vi "PH_Powermeter_BaseClass.set State.vi"(0 "VI in":refnum<vi>, 2 "State":T1, 5 "error in (no error)":errorcluster) -> (14 "VI out":refnum<vi>, 19 "error out":errorcluster)   [LabVIEW 2014, in "PH_Powermeter_BaseClass.lvlib"]
uses:
  PH_Powermeter_BaseClass.lvlib
  PH_Powermeter_BaseClass.State.ctl
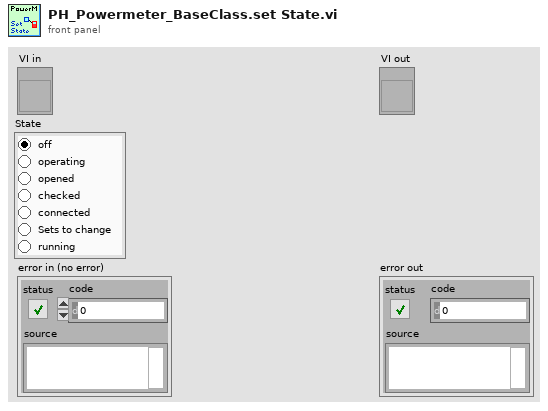
[diagram p1: front panel]
types:
  T1 = typedef "PH_Powermeter_BaseClass.lvlib/PH_Powermeter_BaseClass.State.ctl" = enum32{"off", "operating", "opened", "checked", "connected", "Sets to change", "running"}
  T2 = typedef "PH_Powermeter_BaseClass.lvlib/PH_Powermeter_BaseClass.i attribute.ctl" = cluster{"GUI References":T3, "Connection":T4, "Head Attributes":T5, "VISA resource":refnum<visa-resource-name>, "Energy":T6, "Service ID Energy":i32, "Wanted Settings":T7, "Current Settings":T7}
  T3 = typedef "PH_Powermeter_BaseClass.lvlib/PH_Powermeter_BaseClass.GUI Refs.ctl" = cluster{"Head Attributes":refnum<vi>, "Energy":refnum<vi>, "Connection":refnum<vi>, "VISA Resource":refnum<vi>, "Scaling Factor":refnum<vi>, "Range":refnum<vi>, "Wavelength":refnum<vi>, "Trigger Level":refnum<vi>, "Wanted Settings":refnum<vi>, "Current Settings":refnum<vi>}
  T4 = typedef "PH_Powermeter_BaseClass.lvlib/PH_Powermeter_BaseClass.Connection.ctl" = cluster{"failed checks":i8, "Timeout":bool, "Data read":string, "Failure":bool, "Error":bool, "State":T1}
  T5 = typedef "PH_Powermeter_BaseClass.lvlib/PH_Powermeter_BaseClass.Head Attributes.ctl" = cluster{"Instrument Type":string, "Head Version":string, "Head Name":string, "Serial Number":string, "Firmware":string, "Sensor Type":string, "MinimumRange":u32, "Maximum Range":u32, "Min Wavelength":i32, "Max Wavelength":i32}
  T6 = typedef "PH_Powermeter_BaseClass.lvlib/PH_Powermeter_BaseClass.Energy.ctl" = cluster{"current Value":dbl, "unscaled":dbl, "Scaling Factor":dbl}
  T7 = typedef "PH_Powermeter_BaseClass.lvlib/PH_gentec_BaseClass.Head Settings.ctl" = cluster{"Trigger Level":dbl, "Wavelength":u32, "Range":u32}
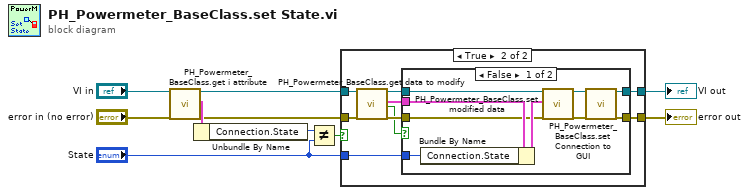
[diagram p0: block diagram]
diagram:
  n1 = call "PH_Powermeter_BaseClass.get i attribute.vi"("i ref in"="VI in", "error in (no error)"="error in (no error)") -> ("i ref out"=w1:refnum<vi>, "i attribute"=w3:T2, "error out"=w2:errorcluster)  [unwired: 15 in]
  n2 = Unbundle By Name(w3) -> ("Connection.State"=w4:T1)
  n3 = Not Equal?(x=w4, y="State") -> (x != y?=w5:bool)
  n4 = case shown="True" w5 {
    tunnel: w1 -> [w12 w17]
    tunnel: w2 -> [w11 w16]
    tunnel: "State" -> [_ w15]
    tunnel: [w12 w14] -> w6
    tunnel: [w11 w13] -> w8
    frame False {
    }
    frame True {
      n5 = call "PH_Powermeter_BaseClass.get data to modify.vi"("i ref in"=w17, "error in (no error)"=w16) -> ("i ref out"=w21:refnum<vi>, "i attribute"=w19:T2, "timed out"=w18:bool, "error out"=w20:errorcluster)  [unwired: 14 in]
      n6 = case shown="False" w18 {
        tunnel: [w24 w32] -> w14
        tunnel: [w22 w31] -> w13
        tunnel: w20 -> [w26 w31]
        tunnel: w21 -> [w30 w32]
        tunnel: w19 -> [w28 _]
        tunnel: w15 -> [w27 _]
        frame False {
          n7 = Bundle By Name(cluster=w28, "Connection.State"=w27) -> (w29:T2)
          n8 = call "PH_Powermeter_BaseClass.set modified data.vi"("i ref in"=w30, "i attribute"=w29, "error in (no error)"=w26) -> ("i ref out"=w25:refnum<vi>, "error out"=w23:errorcluster)  [unwired: 15 in]
          n9 = call "PH_Powermeter_BaseClass.set Connection to GUI.vi"("i ref in"=w25, "error in"=w23) -> ("i ref out"=w24:refnum<vi>, "error out"=w22:errorcluster)  [unwired: 16 in]
        }
        frame True {
        }
      }
    }
  }
  "error out" <- w8
  "VI out" <- w6
